vi "State_Changer.vi"(0 "Action count in":i32[](array[numeric]), 1 "Time in":timestamp, 3 "Action queue in":refnum<queue>, 4 "Current state in":i32, 5 "Current state start in":dbl, 6 "Time of last action in":timestamp[](array[timestamp]), 7 "Abort action":bool, 8 "States":i32[][](array[numeric]), 9 "Actions":i32[][](array[numeric])) -> (10 "Action Queue":i32[](array[numeric]), 12 "Current state index":i32, 13 "Current state start out":dbl, 14 "Action count out":i32[](array[numeric]), 15 "Action Queue out":refnum<queue>, 16 "Time of last action out":timestamp[](array[timestamp]), 17 "Time left":dbl, 18 "Current state out":i32, 19 "error out":errorcluster)   [LabVIEW 2025]
uses:
  TypeDef_State_Action_Columns.ctl
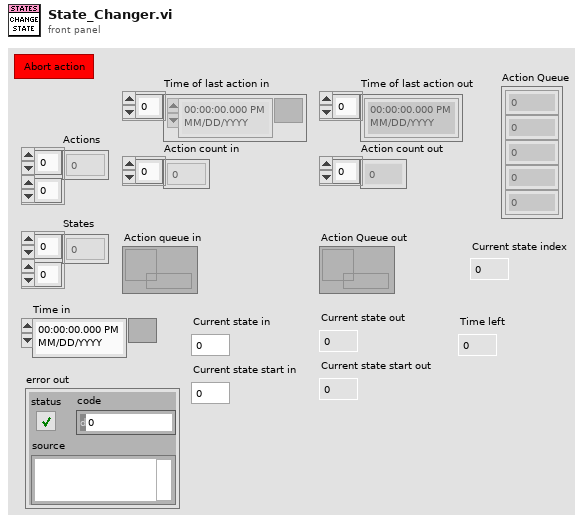
[diagram p1: front panel]
types:
  T1 = typedef "TypeDef_State_Action_Columns.ctl" = enum16{"Action_num", "trigger", "fequency", "offset", "initial state", "mode", "order", "link", "description"}
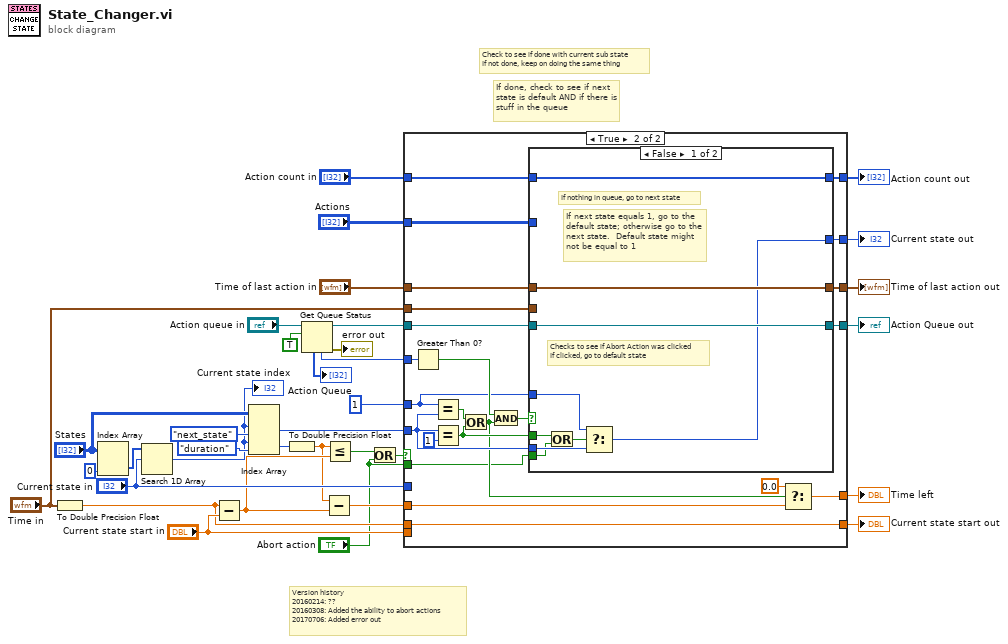
[diagram p0: block diagram]
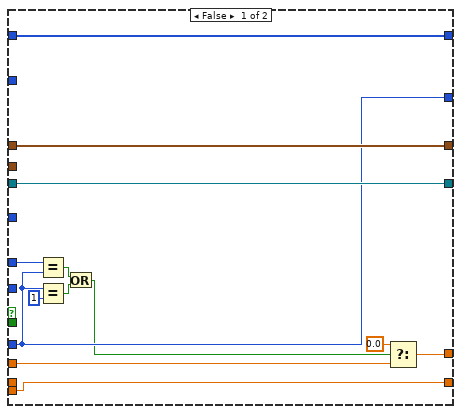
[diagram p2: hidden frame]
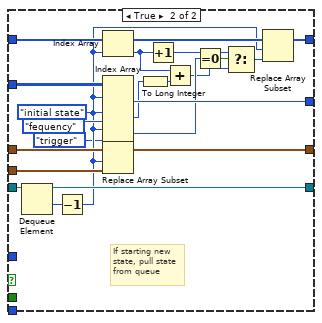
[diagram p3: hidden frame]
diagram:
  # "Version history\n20160214: ??\n20160308: Added the ability to abort actions\n20170706: Added error out"
  # "Check to see if done with current sub state\nIf not done, keep on doing the same thing"
  # "If done, check to see if next state is default AND if there is stuff in the queue"
  n1 = To Double Precision Float(number="Time in") -> (double precision float=w10:dbl)
  n2 = Index Array(array="States", index (col)=0) -> (element=w33:i32[])  [unwired: 1 in]
  n3 = Search 1D Array(1D array=w33, element="Current state in") -> (index of element=w12:i32)  [unwired: 1 in]
  "Current state index" <- w12
  n4 = Subtract(x=w10, y="Current state start in") -> (x-y=w9:dbl)
  n5 = Index Array(array="States", index (row) #1=w12, index (col) #1=enum16{"State_num", "duration", "next_state"}."next_state", index (row) #2=w12, index (col) #2=enum16{"State_num", "duration", "next_state"}."duration") -> (element #1=w14:i32, element #2=w6:i32)
  n6 = To Double Precision Float(number=w6) -> (double precision float=w5:dbl)
  n7 = Get Queue Status(queue="Action queue in", return elements? (F)=TRUE) -> (queue out=w25:refnum<queue>, error out=→"error out":errorcluster, # elements in queue=w16:i32, elements=→"Action Queue":i32[])  [unwired: 1 in, 4 out]
  n8 = Subtract(x=w5, y=w9) -> (x-y=w7:dbl)
  n9 = Less Or Equal?(x=w5, y=w9) -> (x <= y?=w4:bool)
  n10 = Or(x=w4, y="Abort action") -> (x .or. y?=w3:bool)
  n11 = case shown="True" w3 {
    tunnel: w10 -> [_ w66]
    tunnel: "Current state start in" -> [w44 _]
    tunnel: [w44 w66] -> w26
    tunnel: w25 -> [w47 w60]
    tunnel: [w47 w59] -> w24
    tunnel: "Time of last action in" -> [w46 w64]
    tunnel: [w46 w63] -> w21
    tunnel: "Action count in" -> [w45 w62]
    tunnel: [w45 w61] -> w19
    tunnel: "Current state in" -> [w42 _]
    tunnel: [w42 w55] -> w17
    tunnel: w16 -> [_ w70]
    tunnel: 1 ("Default state") -> [w43 w58]
    tunnel: w14 -> [_ w56]
    tunnel: "Actions" -> [_ w54]
    tunnel: "Time in" -> [_ w53]
    tunnel: [w35 w50] -> w8
    tunnel: w7 -> [w37 w49]
    tunnel: "Abort action" -> [_ w48]
    frame False {
      n12 = Equal?(x=w43, y=w42) -> (x = y?=w40:bool)
      n13 = Equal?(x=w42, y=1) -> (x = y?=w39:bool)
      n14 = Or(x=w40, y=w39) -> (x .or. y?=w38:bool)
      n15 = Select(t=0.0, s=w38, f=w37) -> (s? t:f=w35:dbl)
    }
    frame True {
      n16 = Greater Than 0?(x=w70) -> (x > 0?=w67:bool)
      n17 = Equal?(x=w58, y=w56) -> (x = y?=w68:bool)
      n18 = Equal?(x=w56, y=1) -> (x = y?=w57:bool)
      n19 = Or(x=w68, y=w57) -> (x .or. y?=w52:bool)
      n20 = And(x=w67, y=w52) -> (x .and. y?=w65:bool)
      n21 = case shown="False" w65 {
        tunnel: w64 -> [w79 w95]
        tunnel: [w79 w94] -> w63
        tunnel: [w78 w92] -> w61
        tunnel: w62 -> [w78 w91]
        tunnel: w60 -> [w77 w100]
        tunnel: [w77 w99] -> w59
        tunnel: w58 -> [w76 _]
        tunnel: w57 -> [w73 _]
        tunnel: w56 -> [w75 _]
        tunnel: [w74 w96] -> w55
        tunnel: w54 -> [_ w98]
        tunnel: w53 -> [_ w93]
        tunnel: w48 -> [w72 _]
        frame False {
          # "Checks to see if Abort Action was clicked\nIf clicked, go to default state"
          # "If next state equals 1, go to the default state; otherwise go to the next state.  Default state might not be equal to 1"
          # "If nothing in queue, go to next state"
          n22 = Or(x=w73, y=w72) -> (x .or. y?=w71:bool)
          n23 = Select(t=w76, s=w71, f=w75) -> (s? t:f=w74:i32)
        }
        frame True {
          # "If starting new state, pull state from queue"
          n24 = Dequeue Element(queue=w100) -> (queue out=w99:refnum<queue>, element=w101:i32)  [unwired: 2 in, 2 out]
          n25 = Decrement(x=w101) -> (x-1=w86:i32)
          n26 = Index Array(array=w91, index=w86) -> (element=w87:i32)
          n27 = Index Array(array=w98, index (row) #1=w86, index (col) #1=TypeDef_State_Action_Columns."initial state", index (row) #2=w86, index (col) #2=TypeDef_State_Action_Columns."fequency", index (row) #3=w86, index (col) #3=TypeDef_State_Action_Columns."trigger") -> (element #1=w96:i32, element #2=w89:i32, element #3=w84:i32)
          n28 = Replace Array Subset(array=w95, new element=w93, index=w86) -> (w94:timestamp[])
          n29 = To Long Integer(number=w89) -> (32bit integer=w88:i32)
          n30 = Increment(x=w87) -> (x+1=w83:i32)
          n31 = Add(x=w87, y=w88) -> (x+y=w82:i32)
          n32 = Equal To 0?(x=w84) -> (x = 0?=w80:bool)
          n33 = Select(t=w83, s=w80, f=w82) -> (s? t:f=w81:i32)
          n34 = Replace Array Subset(array=w91, new element=w81, index=w86) -> (w92:i32[])
        }
      }
      n35 = Select(t=0.0, s=w52, f=w49) -> (s? t:f=w50:dbl)
    }
  }
  "Action Queue out" <- w24
  "Current state out" <- w17
  "Current state start out" <- w26
  "Time of last action out" <- w21
  "Action count out" <- w19
  "Time left" <- w8
